vi "Factorial of numbers without uing shift registers in LabVIEW.vi"() -> ()   [LabVIEW 2026]
panel:
  out "INPUT":dbl
  out "INPUT":dbl
  # "WHILE loop"
  # "FOR loop"
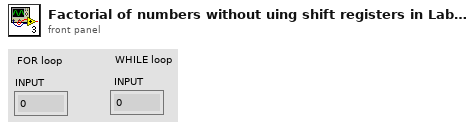
[diagram p1: front panel]
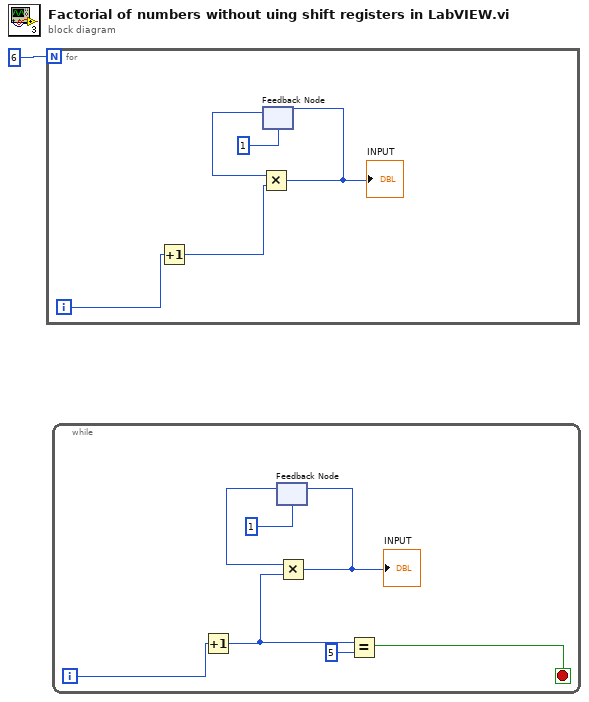
[diagram p0: block diagram]
diagram:
  n1 = for {
    N: 6 ("Numeric") -> [_]
    i -> [w5]
    n2 = Increment(x=w5) -> (x+1=w4:i32)
    n3 = feedback #1(1) -> (w6:i32)
    n4 = Multiply(x=w6, y=w4) -> (x*y=w3:i32)
    "INPUT" <- w3
    n5 = feedback-in #1(w3) -> ()
  }
  n6 = while {
    i -> [w13]
    stop <- w7 stop-if-true
    n7 = Increment(x=w13) -> (x+1=w9:i32)
    n8 = feedback #2(1) -> (w12:i32)
    n9 = Multiply(x=w12, y=w9) -> (x*y=w11:i32)
    "INPUT" <- w11
    n10 = feedback-in #2(w11) -> ()
    n11 = Equal?(x=w9, y=5) -> (x = y?=w7:bool)
  }
